vi "GetVessels.vi"(8 "error in (no error)":errorcluster, 9 "Position":dbl[](array[numeric]), 10 "condition":string, 11 "Database in":refnum<class "Database.lvclass">) -> (0 "error out":errorcluster, 2 "Vessel Cluster":T1, 3 "Database out":refnum<class "Database.lvclass">)   [LabVIEW 2012, in "Database.lvclass"]
uses:
  Database.lvclass
  Database.lvclass/Database.ctl
  <vilib>/addons/database/_DB Variant To Data/Database Variant To Data.xnode
  <vilib>/addons/database/NI_Database_API.lvlib
panel:
  out "looking for file:":path
  in  "Default Pos":dbl[](array[numeric])
  in  "Cluster":T1
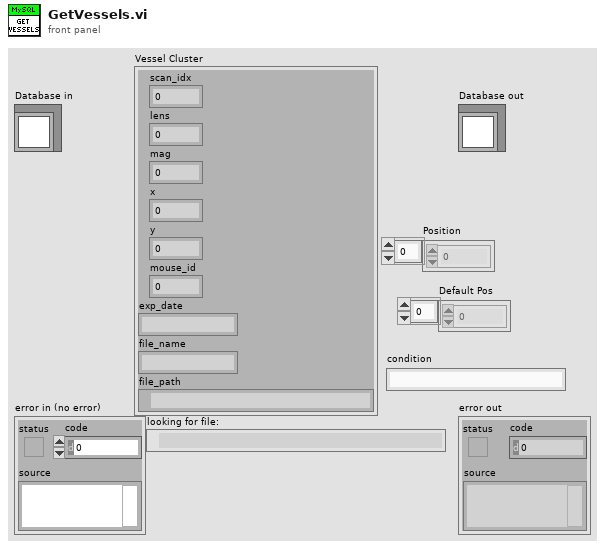
[diagram p1: front panel]
types:
  T1 = cluster{"scan_idx":i32, "lens":i32, "mag":dbl, "x":dbl, "y":dbl, "mouse_id":i32, "exp_date":string, "file_name":string, "file_path":path}
  T2 = typedef "NI_Database_API.lvlib/Conn ObjectReference.ctl" = refnum<k1>
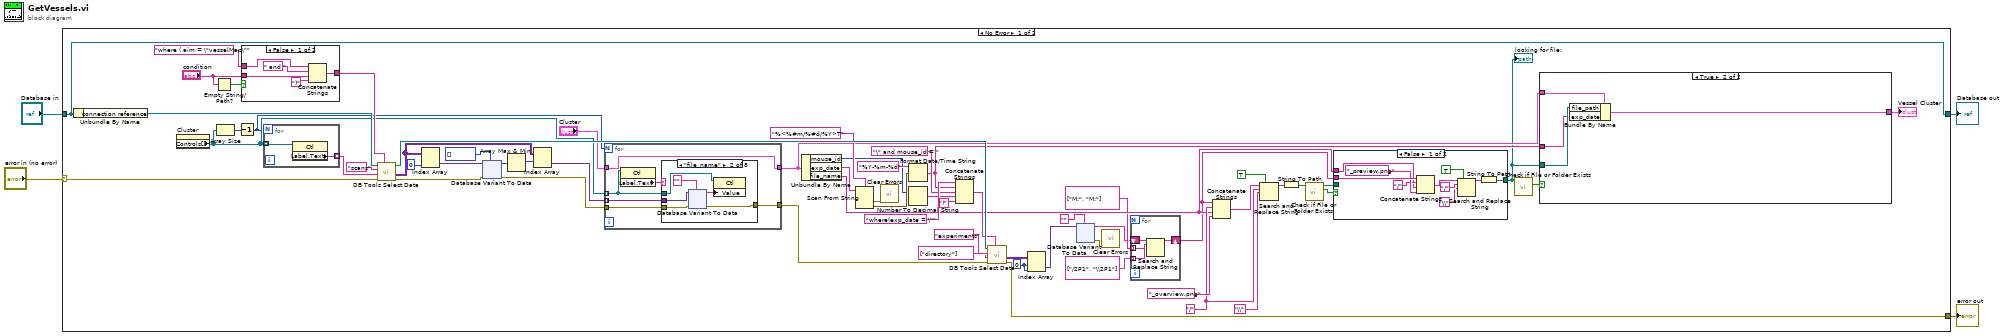
[diagram p0: block diagram]
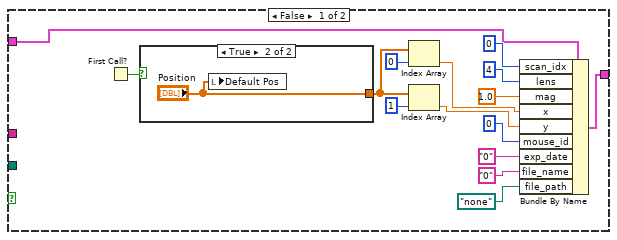
[diagram p3: hidden frame]
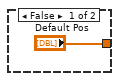
[diagram p4: hidden frame]
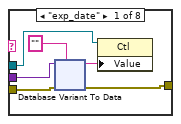
[diagram p5: hidden frame]
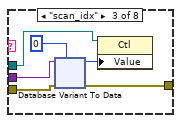
[diagram p6: hidden frame]
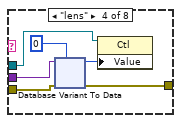
[diagram p7: hidden frame]
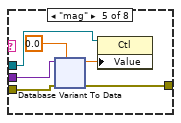
[diagram p8: hidden frame]
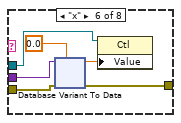
[diagram p9: hidden frame]
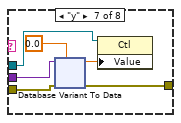
[diagram p10: hidden frame]
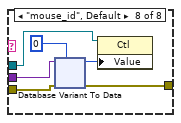
[diagram p11: hidden frame]
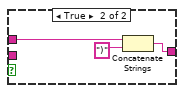
[diagram p12: hidden frame]
diagram:
  n1 = case shown="No Error" "error in (no error)" {
    selector: "error in (no error)" -> [w54 w494]
    tunnel: [w20 w494] -> w3
    tunnel: [w65 w493] -> w1
    tunnel: "Database in" -> [w65 w493]
    frame No Error {
      w11 = "/" ("search string")
      w37 = 0 ("index (row)")
      n2 = Unbundle By Name(w65) -> ("connection reference"=w64:T2)
      n3 = property on="Cluster" class="Clust (strict)"() -> ("Controls[]"=w52:refnum<vi>[])  [unwired: 2 in, 2 out]
      n4 = Empty String/Path?(string/path="condition") -> (empty?=w62:bool)
      n5 = Array Size(array=w52) -> (size(s)=w57:i32)
      n6 = Decrement(x=w57) -> (x-1=w51:i32)
      n7 = case shown="False" w62 {
        tunnel: "where ( aim = \"vesselMap\"" ("condition") -> [w489 w491]
        tunnel: [w485 w490] -> w60
        tunnel: "condition" -> [w487 _]
        frame False {
          n8 = Concatenate Strings(w489, " and ", w487, ")" ("string")) -> (w485:string)
        }
        frame True {
          n9 = Concatenate Strings(w491, ")" ("string")) -> (w490:string)
        }
      }
      n10 = for {
        N: w51 -> [_]
        tunnel: w52 -> [w484] mode=indexing
        tunnel: [w483] -> w55 mode=indexing
        n11 = property class="Ctl"(reference=w484) -> ("Label.Text"=w483:string)  [unwired: 1 in, 2 out]
      }
      n12 = call <vilib>:"DB Tools Select Data.vi"("condition"=w60, "error in (no error)"=w54, "columns"=w55, "table"="scans", "connection reference"=w64) -> ("error out"=w50:errorcluster, "data"=w56:variant[][], "connection reference out"=w58:T2)  [unwired: 1 in]
      n13 = Index Array(array=w56, index (col)=0 ("disabled index (col)")) -> (element=w48:variant[])  [unwired: 1 in]
      n14 = xnode "Database Variant To Data"("database variant"=w48, "error in"=w50, "type"=i32[] []) -> ("data"=w46:i32[], "error out"=w25:errorcluster)
      n15 = Array Max & Min(array=w46) -> (max index (indices)=w31:i32)  [unwired: 3 out]
      n16 = Index Array(array=w56, index (row)=w31) -> (element=w30:variant[])  [unwired: 1 in]
      n17 = for {
        N: w51 -> [_]
        tunnel: w52 -> [w105] mode=indexing
        tunnel: w30 -> [w108] mode=indexing
        tunnel: "Cluster" -> [w107]
        tunnel: [w107] -> w27
        tunnel: w25 -> [w104]
        tunnel: [w103] -> w24
        n18 = property class="Ctl"(reference=w105) -> ("Label.Text"=w106:string)  [unwired: 1 in, 2 out]
        n19 = case shown="\"file_name\"" w106 {
          tunnel: w108 -> [w114 w151 w188 w225 w263 w301 w340 w378]
          tunnel: w105 -> [w113 w149 w189 w226 w264 w302 w339 w377]
          tunnel: w104 -> [w110 w148 w186 w224 w262 w300 w338 w376]
          tunnel: [w109 w147 w185 w223 w261 w299 w337 w375] -> w103
          frame "exp_date" {
            n20 = xnode "Database Variant To Data"("database variant"=w114, "error in"=w110, "type"="") -> ("data"=w111:string, "error out"=w109:errorcluster)
            n21 = property class="Ctl"(reference=w113, "Value"=w111) -> ()  [unwired: 1 in, 2 out]
          }
          frame "file_name" {
            n22 = xnode "Database Variant To Data"("database variant"=w151, "error in"=w148, "type"="") -> ("data"=w152:string, "error out"=w147:errorcluster)
            n23 = property class="Ctl"(reference=w149, "Value"=w152) -> ()  [unwired: 1 in, 2 out]
          }
          frame "scan_idx" {
            n24 = xnode "Database Variant To Data"("database variant"=w188, "error in"=w186, "type"=0) -> ("data"=w190:i32, "error out"=w185:errorcluster)
            n25 = property class="Ctl"(reference=w189, "Value"=w190) -> ()  [unwired: 1 in, 2 out]
          }
          frame "lens" {
            n26 = xnode "Database Variant To Data"("database variant"=w225, "error in"=w224, "type"=0) -> ("data"=w228:i32, "error out"=w223:errorcluster)
            n27 = property class="Ctl"(reference=w226, "Value"=w228) -> ()  [unwired: 1 in, 2 out]
          }
          frame "mag" {
            n28 = xnode "Database Variant To Data"("database variant"=w263, "error in"=w262, "type"=0.0) -> ("data"=w266:dbl, "error out"=w261:errorcluster)
            n29 = property class="Ctl"(reference=w264, "Value"=w266) -> ()  [unwired: 1 in, 2 out]
          }
          frame "x" {
            n30 = xnode "Database Variant To Data"("database variant"=w301, "error in"=w300, "type"=0.0) -> ("data"=w304:dbl, "error out"=w299:errorcluster)
            n31 = property class="Ctl"(reference=w302, "Value"=w304) -> ()  [unwired: 1 in, 2 out]
          }
          frame "y" {
            n32 = xnode "Database Variant To Data"("database variant"=w340, "error in"=w338, "type"=0.0) -> ("data"=w342:dbl, "error out"=w337:errorcluster)
            n33 = property class="Ctl"(reference=w339, "Value"=w342) -> ()  [unwired: 1 in, 2 out]
          }
          frame "mouse_id", Default {
            n34 = xnode "Database Variant To Data"("database variant"=w378, "error in"=w376, "type"=i16 0) -> ("data"=w380:i16, "error out"=w375:errorcluster)
            n35 = property class="Ctl"(reference=w377, "Value"=w380) -> ()  [unwired: 1 in, 2 out]
          }
        }
      }
      n36 = Unbundle By Name(w27) -> ("mouse_id"=w29:i32, "exp_date"=w28:string, "file_name"=w10:string)
      n37 = Scan From String(format string="%<%#m/%#d/%Y>T" ("input string"), input string=w28) -> (error out=w21:errorcluster, output 1=w33:timestamp)  [unwired: 2 in, 3 out]
      n38 = call <vilib>:"Clear Errors.vi"("error in (no error)"=w21) -> ()  [unwired: 6 in, 1 out]
      n39 = Format Date/Time String(time format string (%c)="%Y-%m-%d", seconds (now)=w33) -> (date/time string=w26:string)  [unwired: 1 in]
      n40 = Number To Decimal String(number=w29) -> (decimal integer string=w40:string)  [unwired: 1 in]
      n41 = Concatenate Strings("where(exp_date = \"" ("string"), w26, "\" and mouse_id = " ("string"), w40, ")" ("string")) -> (w39:string)
      n42 = call <vilib>:"DB Tools Select Data.vi"("condition"=w39, "error in (no error)"=w24, "columns"=string[] ["directory"], "table"="experiments", "connection reference"=w58) -> ("error out"=w20:errorcluster, "data"=w38:variant[][])  [unwired: 1 in, 1 out]
      n43 = Index Array(array=w38, index (row)=w37, index (col)=w37) -> (element=w36:variant)
      n44 = xnode "Database Variant To Data"("database variant"=w36, "type"="") -> ("data"=w6:string, "error out"=w19:errorcluster)  [unwired: 1 in]
      n45 = call <vilib>:"Clear Errors.vi"("error in (no error)"=w19) -> ()  [unwired: 6 in, 1 out]
      n46 = for {
        tunnel: string[] ["M:", "M:"] -> [w67] mode=indexing
        tunnel: string[] ["/2P1", "\\2P1"] -> [w68] mode=indexing
        shift-right: [w69] -> w5
        shift-left: w6 -> [w70]
        n47 = Search and Replace String(input string=w70, search string=w68, replace string=w67) -> (result string=w69:string)  [unwired: 5 in, 3 out]
      }
      n48 = Concatenate Strings(w5, w11, w10, "_overview.png" ("string")) -> (w14:string)
      n49 = Search and Replace String(replace all?=TRUE ("replace all? (F)"), input string=w14, search string=w11, replace string="\\" ("replace string (\"\")")) -> (result string=w16:string)  [unwired: 4 in, 3 out]
      n50 = String To Path(string=w16) -> (path=w18:path)
      n51 = call <vilib>:"Check if File or Folder Exists.vi"("path"=w18) -> ("file or folder exists?"=w12:bool, "dup path"=w9:path)  [unwired: 8 in, 1 out]
      n52 = case shown="False" w12 {
        tunnel: w5 -> [w80 _]
        tunnel: w10 -> [w72 _]
        tunnel: [w71 w81] -> w23
        tunnel: w9 -> [_ w81]
        frame False {
          n53 = Concatenate Strings(w80, "/" ("string"), w72, "_preview.png" ("string")) -> (w77:string)
          n54 = Search and Replace String(replace all?=TRUE ("replace all? (F)"), input string=w77, search string="/", replace string="\\" ("replace string (\"\")")) -> (result string=w74:string)  [unwired: 4 in, 3 out]
          n55 = String To Path(string=w74) -> (path=w71:path)
        }
        frame True {
        }
      }
      "looking for file:" <- w23
      n56 = call <vilib>:"Check if File or Folder Exists.vi"("path"=w23) -> ("file or folder exists?"=w22:bool)  [unwired: 8 in, 2 out]
      n57 = case shown="True" w22 {
        tunnel: [w90 w102] -> w49
        tunnel: w23 -> [_ w101]
        tunnel: w27 -> [w89 w100]
        tunnel: w26 -> [_ w99]
        frame False {
          n58 = First Call?() -> (First Call?: T/F=w82:bool)
          n59 = case shown="True" w82 {
            tunnel: ["Default Pos" "Position"] -> w87
            frame False {
            }
            frame True {
              n60 = local write "Default Pos"("Position") -> ()
            }
          }
          n61 = Index Array(array=w87, index=0) -> (element=w84:dbl)
          n62 = Index Array(array=w87, index=1) -> (element=w83:dbl)
          n63 = Bundle By Name(cluster=w89, "scan_idx"=0, "lens"=4, "mag"=1.0, "x"=w84, "y"=w83, "mouse_id"=0, "exp_date"="0", "file_name"="0", "file_path"=path "none") -> (w90:T1)
        }
        frame True {
          n64 = Bundle By Name(cluster=w100, "file_path"=w101, "exp_date"=w99) -> (w102:T1)
        }
      }
      "Vessel Cluster" <- w49
    }
    frame Error {
    }
  }
  "error out" <- w3
  "Database out" <- w1
